vi "Reproductord.vi"() -> ()   [LabVIEW 2017]
uses:
  <vilib>/sound2/lvsound2.llb/Sound File Position.ctl
  <vilib>/Analysis/baseanly.llb/Mean (DBL).vi
  <vilib>/sound2/lvsound2.llb/Sound File Read (DBL).vi
  <vilib>/measure/matone.llb/Extract Single Tone Information N Chan.vi
  <vilib>/measure/maspectr.llb/FFT Spectrum (Mag-Phase) for N Chan.vi
  <vilib>/sound2/lvsound2.llb/Sound Output Write (DBL).vi
  <vilib>/measure/NI_MAPro.lvlib
  <vilib>/Analysis/NI_AALBase.lvlib
panel:
  out "Escala":picture
  out "Cancion":waveform(dbl)[](graph)
  out "FFT":cluster{"f0":dbl, "df":dbl, "magnitude":dbl[]}[](graph)
  out "Array":path[](array[path])
  out "filenames":string[](array[string])
  in  "Skip Forward Button":bool
  in  "Skip Back Button":bool
  in  "Seek Forward Button":bool
  in  "Seek Back Button":bool
  in  "Media Stop Button":bool
  in  "Pause Button":bool
  in  "Play Button":bool
  in  "stop":bool
  in  "path":path
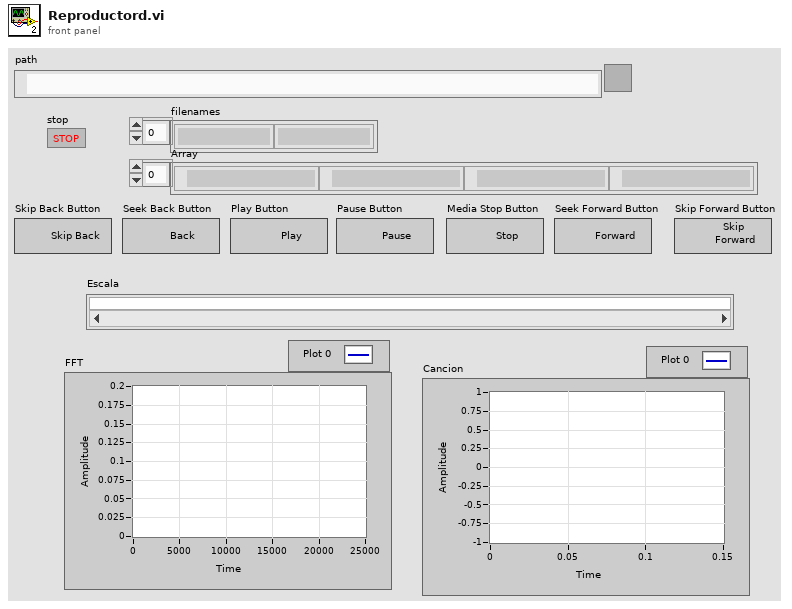
[diagram p1: front panel]
types:
  T1 = typedef "imagedata.ctl" = cluster{"image type":i32, "image depth":i32, "image":u8[], "mask":u8[], "colors":u32[], "Rectangle":cluster{"left":i16, "top":i16, "right":i16, "bottom":i16}}
  T2 = typedef "Sound Output Task ID.ctl" = u32
  T3 = typedef "Sound File Refnum.ctl" = refnum<file>
  T4 = cluster{"sound file refnum out":T3, "Error_A":errorcluster, "task ID out":T2, "Error_B":errorcluster, "Indice":i32, "Reproduccion":i32, "Numero de Cancion":i32}
  T5 = typedef "Sound File Position.ctl" = u16
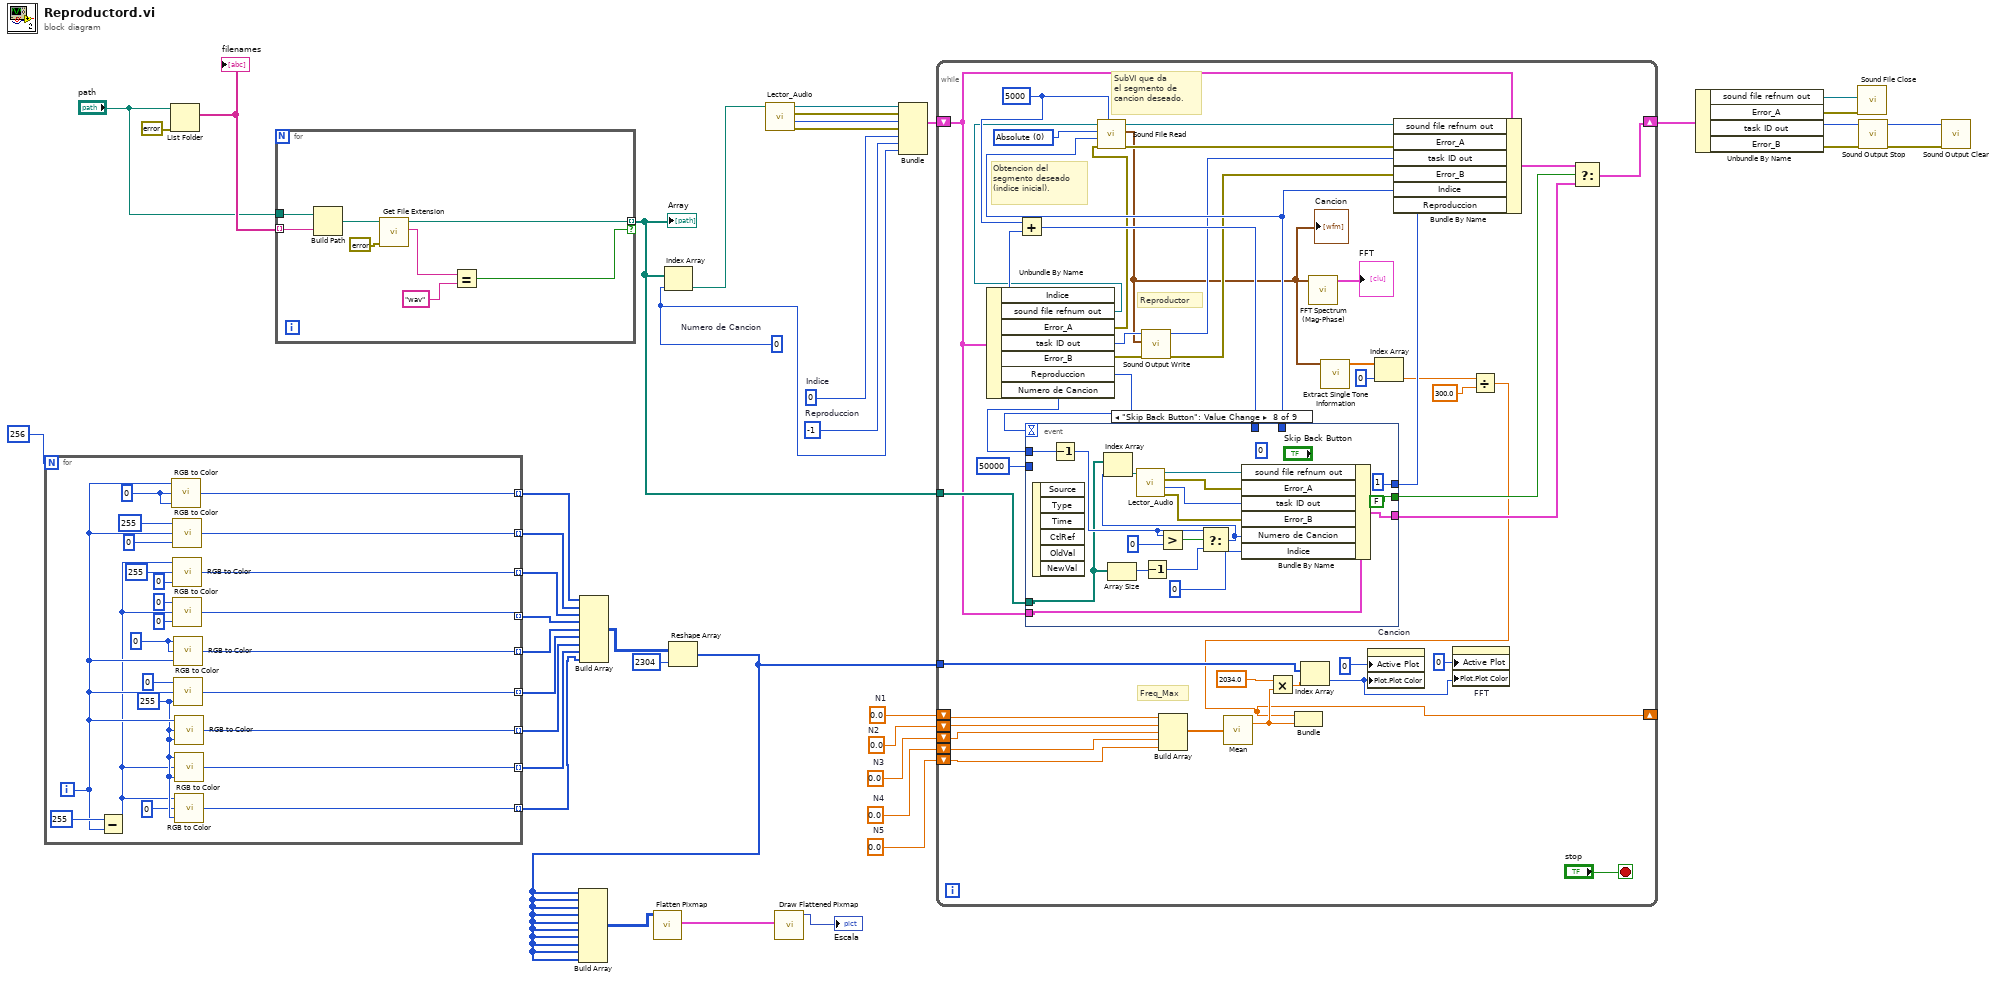
[diagram p0: block diagram]
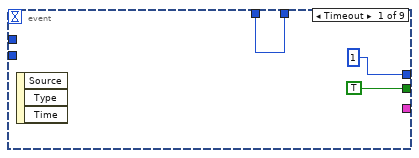
[diagram p2: hidden frame]
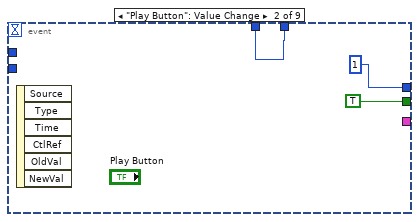
[diagram p3: hidden frame]
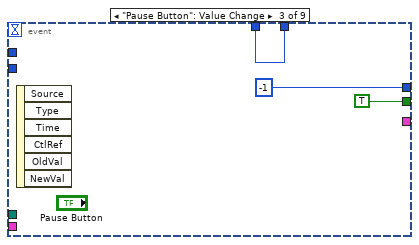
[diagram p4: hidden frame]
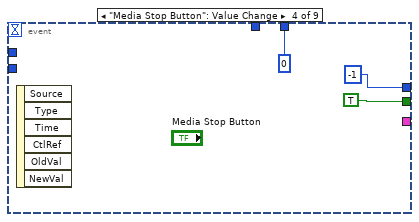
[diagram p5: hidden frame]
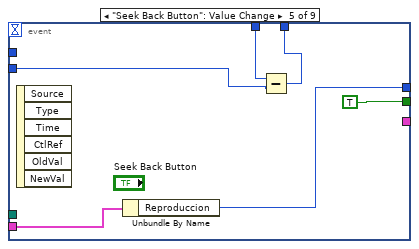
[diagram p6: hidden frame]
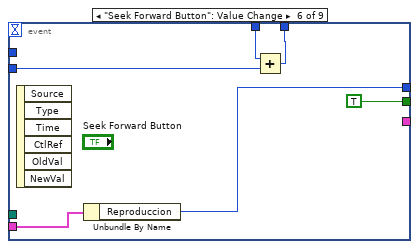
[diagram p7: hidden frame]
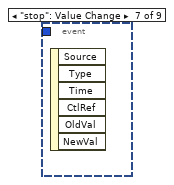
[diagram p8: hidden frame]
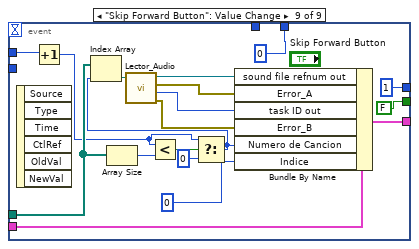
[diagram p9: hidden frame]
diagram:
  w1 = 0.0  # N5
  w2 = 0.0  # N4
  w3 = 0.0  # N3
  w4 = 0.0  # N2
  w5 = 0.0  # N1
  w28 = 0  # Numero de Cancion
  w32 = -1  # Reproduccion
  w33 = 0  # Indice
  n1 = for {
    N: 256 -> [_]
    tunnel: [w64] -> w11 mode=indexing
    tunnel: [w63] -> w10 mode=indexing
    tunnel: [w62] -> w20 mode=indexing
    tunnel: [w61] -> w19 mode=indexing
    tunnel: [w60] -> w18 mode=indexing
    tunnel: [w59] -> w17 mode=indexing
    tunnel: [w58] -> w16 mode=indexing
    tunnel: [w57] -> w15 mode=indexing
    tunnel: [w56] -> w14 mode=indexing
    i -> [w45]
    w44 = u8 255 ("B")
    w48 = u8 0 ("R")
    w47 = u8 0 ("G")
    n2 = Subtract(x=255, y=w45) -> (x-y=w42:i32)
    n3 = call <vilib>:"RGB to Color.vi"("B"=w47, "G"=w47, "R"=w45) -> ("Color"=w64:u32)
    n4 = call <vilib>:"RGB to Color.vi"("B"=u8 0, "G"=w45, "R"=u8 255) -> ("Color"=w63:u32)
    n5 = call <vilib>:"RGB to Color.vi"("B"=u8 0, "G"=u8 255, "R"=w42) -> ("Color"=w62:u32)
    n6 = call <vilib>:"RGB to Color.vi"("B"=u8 0, "G"=w42, "R"=u8 0) -> ("Color"=w61:u32)
    n7 = call <vilib>:"RGB to Color.vi"("B"=w45, "G"=w48, "R"=w48) -> ("Color"=w60:u32)
    n8 = call <vilib>:"RGB to Color.vi"("B"=w44, "G"=w45, "R"=u8 0 ("G")) -> ("Color"=w59:u32)
    n9 = call <vilib>:"RGB to Color.vi"("B"=w44, "G"=w44, "R"=w45) -> ("Color"=w58:u32)
    n10 = call <vilib>:"RGB to Color.vi"("B"=w44, "G"=w42, "R"=w44) -> ("Color"=w57:u32)
    n11 = call <vilib>:"RGB to Color.vi"("B"=w44, "G"=u8 0 ("R"), "R"=w42) -> ("Color"=w56:u32)
  }
  n12 = List Folder(path="path", error in=errorcluster {"status"=FALSE, "code"=0, "source"=""}) -> (filenames=w30:string[])  [unwired: 2 in, 3 out]
  "filenames" <- w30
  n13 = for {
    tunnel: w30 -> [w72] mode=indexing
    tunnel: "path" -> [w71]
    tunnel: [w66] -> w27 mode=indexing if=w65
    n14 = Build Path(base path=w71, name or relative path=w72) -> (appended path=w70:path)
    n15 = call <vilib>:"Get File Extension.vi"("error in (no error)"=errorcluster {"status"=FALSE, "code"=0, "source"=""}, "file"=w70) -> ("lowercase file extension"=w68:string, "dup file"=w66:path)  [unwired: 5 in, 3 out]
    n16 = Equal?(x=w68, y="wav") -> (x = y?=w65:bool)
  }
  "Array" <- w27
  n17 = Build Array "Build Array"(w11, w10, w20, w19, w18, w17, w16, w15, w14) -> (w13:u32[][])
  n18 = Index Array "Index Array"(array=w27, index=w28) -> (element=w26:path)
  n19 = Reshape Array(w13, 2304 ("dimension size")) -> (w6:u32[])
  n20 = Build Array(w6, w6, w6, w6, w6, w6, w6, w6, w6, w6) -> (w7:u32[][])
  n21 = call <vilib>:"Flatten Pixmap.vi"("24-bit pixmap"=w7) -> ("image data"=w9:T1)  [unwired: 10 in]
  n22 = call "Lector_Audio.vi"("path"=w26) -> ("Error_B"=w22:errorcluster, "task ID out"=w23:T2, "Error_A"=w24:errorcluster, "sound file refnum out"=w25:T3)  [unwired: 7 in]
  n23 = call <vilib>:"Draw Flattened Pixmap.vi"("image data"=w9) -> ("new picture"=→"Escala":picture)  [unwired: 8 in]
  n24 = Bundle("sound file refnum out"=w25, "Error_A"=w24, "task ID out"=w23, "Error_B"=w22, "Indice"=w33, "Reproduccion"=w32, "Numero de Cancion"=w28) -> (w39:T4)  [unwired: 1 in]
  n25 = while {
    shift-right: [w97] -> w38
    shift-left: w39 -> [w96]
    tunnel: w27 -> [w106]
    tunnel: w6 -> [w87]
    shift-right: [w75] -> _
    shift-left: w5 -> [w86]
    shift-left: w4 -> [w85]
    shift-left: w3 -> [w84]
    shift-left: w2 -> [w83]
    shift-left: w1 -> [w82]
    stop <- "stop" stop-if-true
    w113 = 5000 ("number of samples/ch (-1: all)")
    w116 = T5 0 items=["Absolute"=0, "Relative"=2] ("position mode")
    # "Freq_Max"
    # "SubVI que da\nel segmento de\ncancion deseado."
    # "Reproductor"
    # "Obtencion del \nsegmento deseado\n(indice inicial)."
    n26 = Unbundle By Name(w96) -> ("Indice"=w114:i32, "sound file refnum out"=w103:T3, "Error_A"=w102:errorcluster, "task ID out"=w104:T2, "Error_B"=w105:errorcluster, "Reproduccion"=w109:i32, "Numero de Cancion"=w107:i32)
    n27 = Add(x=w113, y=w114) -> (x+y=w112:i32)
    n28 = event shown="[7] \"Skip Back Button\": Value Change" {
      selector: _ -> [_ _ _ _ _ _ _ _ _]
      dyn-events: _ -> [_ _ _ _ _ _ _ _ _]
      timeout: w109 -> [_ _ _ _ _ _ _ _ _]
      tunnel: w112 -> [w119 w121 w124 _ w134 w139 _ _ _]
      tunnel: [w119 w121 w124 0 w133 w138 _ _ 0] -> w111
      tunnel: [1 1 -1 -1 w129 w135 _ 1 1] -> w110
      tunnel: 50000 ("y") -> [_ _ _ _ w132 w140 _ _ _]
      tunnel: w107 -> [_ _ _ _ _ _ _ w145 w176]
      tunnel: w106 -> [_ _ _ _ _ _ _ w143 w165]
      tunnel: w96 -> [_ _ _ _ w130 w136 _ w149 w174]
      tunnel: [_ _ _ _ _ _ _ w148 w168] -> w95
      tunnel: [TRUE TRUE TRUE TRUE TRUE TRUE _ FALSE FALSE] -> w94
      event Timeout {
        n29 = event-data() -> ()  [unwired: 1 in, 3 out]
      }
      event "Play Button": Value Change {
        n30 = event-data() -> ()  [unwired: 1 in, 6 out]
      }
      event "Pause Button": Value Change {
        n31 = event-data() -> ()  [unwired: 1 in, 6 out]
      }
      event "Media Stop Button": Value Change {
        n32 = event-data() -> ()  [unwired: 1 in, 6 out]
      }
      event "Seek Back Button": Value Change {
        n33 = event-data() -> ()  [unwired: 1 in, 6 out]
        n34 = Unbundle By Name(w130) -> ("Reproduccion"=w129:i32)
        n35 = Subtract(x=w134, y=w132) -> (x-y=w133:i32)
      }
      event "Seek Forward Button": Value Change {
        n36 = event-data() -> ()  [unwired: 1 in, 6 out]
        n37 = Unbundle By Name(w136) -> ("Reproduccion"=w135:i32)
        n38 = Add(x=w139, y=w140) -> (x+y=w138:i32)
      }
      event "stop": Value Change {
        n39 = event-data() -> ()  [unwired: 1 in, 6 out]
      }
      event "Skip Back Button": Value Change {
        (unwired) 0
        n40 = event-data() -> ()  [unwired: 1 in, 6 out]
        n41 = Decrement(x=w145) -> (x-1=w152:i32)
        n42 = Array Size(array=w143) -> (size(s)=w142:i32)
        n43 = Decrement(x=w142) -> (x-1=w141:i32)
        n44 = Greater?(x=w152, y=0 ("f")) -> (0:w153:bool)
        n45 = Select(t=w152, s=w153, f=w141) -> (s? t:f=w151:i32)
        n46 = Index Array(array=w143, index=w151) -> (element=w158:path)
        n47 = call "Lector_Audio.vi"("path"=w158) -> ("Error_B"=w154:errorcluster, "task ID out"=w155:T2, "Error_A"=w156:errorcluster, "sound file refnum out"=w157:T3)  [unwired: 7 in]
        n48 = Bundle By Name(cluster=w149, "sound file refnum out"=w157, "Error_A"=w156, "task ID out"=w155, "Error_B"=w154, "Numero de Cancion"=w151, "Indice"=0) -> (w148:T4)
      }
      event "Skip Forward Button": Value Change {
        n49 = event-data() -> ()  [unwired: 1 in, 6 out]
        n50 = Increment(x=w176) -> (x+1=w162:i32)
        n51 = Array Size(array=w165) -> (size(s)=w164:i32)
        n52 = Less?(x=w162, y=w164) -> (x < y?=w163:bool)
        n53 = Select(t=w162, s=w163, f=0) -> (s? t:f=w160:i32)
        n54 = Index Array(array=w165, index=w160) -> (element=w175:path)
        n55 = call "Lector_Audio.vi"("path"=w175) -> ("Error_B"=w170:errorcluster, "task ID out"=w171:T2, "Error_A"=w172:errorcluster, "sound file refnum out"=w173:T3)  [unwired: 7 in]
        n56 = Bundle By Name(cluster=w174, "sound file refnum out"=w173, "Error_A"=w172, "task ID out"=w171, "Error_B"=w170, "Numero de Cancion"=w160, "Indice"=0) -> (w168:T4)
      }
    }
    n57 = call-poly <vilib>:"Sound File Read.vi"("number of samples/ch (-1: all)"=w113, "error in (no error)"=w102, "position offset"=w111, "position mode"=w116, "sound file refnum"=w103) -> ("error out"=w101:errorcluster, "data"=w80:waveform(dbl)[], "sound file refnum out"=w93:T3)  [unwired: 2 in, 2 out]
    "Cancion" <- w80
    n58 = call-poly <vilib>:"Sound Output Write.vi"("error in (no error)"=w105, "data"=w80, "task ID"=w104) -> ("error out"=w99:errorcluster, "task ID out"=w100:T2)  [unwired: 7 in]
    n59 = Build Array(w86, w85, w84, w83, w82) -> (w91:dbl[])
    n60 = call-poly <vilib>:"Mean.vi"("X"=w91) -> ("mean"=w88:dbl)  [unwired: 1 out]
    n61 = Multiply(x=2034.0, y=w88) -> (x*y=w89:dbl)
    n62 = Index Array(array=w87, index=w89) -> (element=w74:u32)
    n63 = call-poly <vilib>:"FFT Spectrum (Mag-Phase).vi"("time signals"=w80) -> ("magnitudes"=→"FFT":cluster{"f0":dbl, "df":dbl, "magnitude":dbl[]}[])  [unwired: 6 in, 4 out]
    n64 = call-poly <vilib>:"Extract Single Tone Information.vi"("time signals in"=w80) -> ("detected frequencies"=w79:dbl[])  [unwired: 5 in, 5 out]
    n65 = property on="Cancion" class="WFGraph (strict)"("Active Plot"=0, "Plot.Plot Color"=w74) -> ()  [unwired: 2 in, 2 out]
    n66 = Index Array(array=w79, index=0) -> (element=w77:dbl)
    n67 = Bundle By Name(cluster=w96, "sound file refnum out"=w93, "Error_A"=w101, "task ID out"=w100, "Error_B"=w99, "Indice"=w111, "Reproduccion"=w110) -> (w98:T4)
    n68 = property on="FFT" class="WFGraph (strict)"("Active Plot"=u32 0, "Plot.Plot Color"=w74) -> ()  [unwired: 2 in, 2 out]
    n69 = Divide(x=w77, y=300.0) -> (x/y=w75:dbl)
    n70 = Bundle(w75, "mean"=w88) -> ()  [unwired: 1 in, 1 out]
    n71 = Select(t=w98, s=w94, f=w95) -> (s? t:f=w97:T4)
  }
  n72 = Unbundle By Name(w38) -> ("sound file refnum out"=w37:T3, "Error_A"=w36:errorcluster, "task ID out"=w35:T2, "Error_B"=w34:errorcluster)
  n73 = call <vilib>:"Sound File Close.vi"("error in (no error)"=w36, "sound file refnum"=w37) -> ()  [unwired: 9 in, 1 out]
  n74 = call <vilib>:"Sound Output Stop.vi"("error in (no error)"=w34, "task ID"=w35) -> ("error out"=w40:errorcluster, "task ID out"=w41:T2)  [unwired: 8 in]
  n75 = call <vilib>:"Sound Output Clear.vi"("error in (no error)"=w40, "task ID"=w41) -> ()  [unwired: 9 in, 1 out]
